vi "oldDataToTDMS.vi"() -> ()   [LabVIEW 2018]
uses:
  PublicSubVI/Class/FileManager/FM.lvclass
  PublicSubVI/Class/ProgressBar/ProgressBar.lvclass
panel:
  in  "Progress":i32(slide) caption="AddPath" scale=0.0..100.0
  out "conversion failure path list":i32(listbox)=-1
  in  "progressCaption":string
  in  "conversion":bool
  in  "path list":i32(listbox)=-1
  in  "add data path":path
  in  "target folder path ( TDMS )":path
  in  "reset":bool
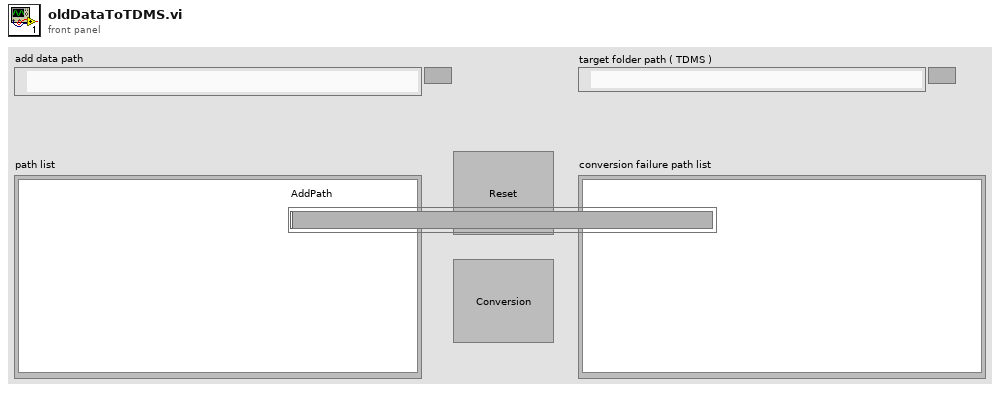
[diagram p1: front panel]
types:
  T1 = cluster{"thisVIRefnum":refnum<vi>, "progressBarRefnum":refnum<vi>, "progressCaption":refnum<vi>}
  T2 = enum16{"open", "open or create", "create or replace", "create", "open (read-only)"}
  T3 = enum16{"open", "replace", "create", "open or create", "replace or create", "replace or create with confirmation"}
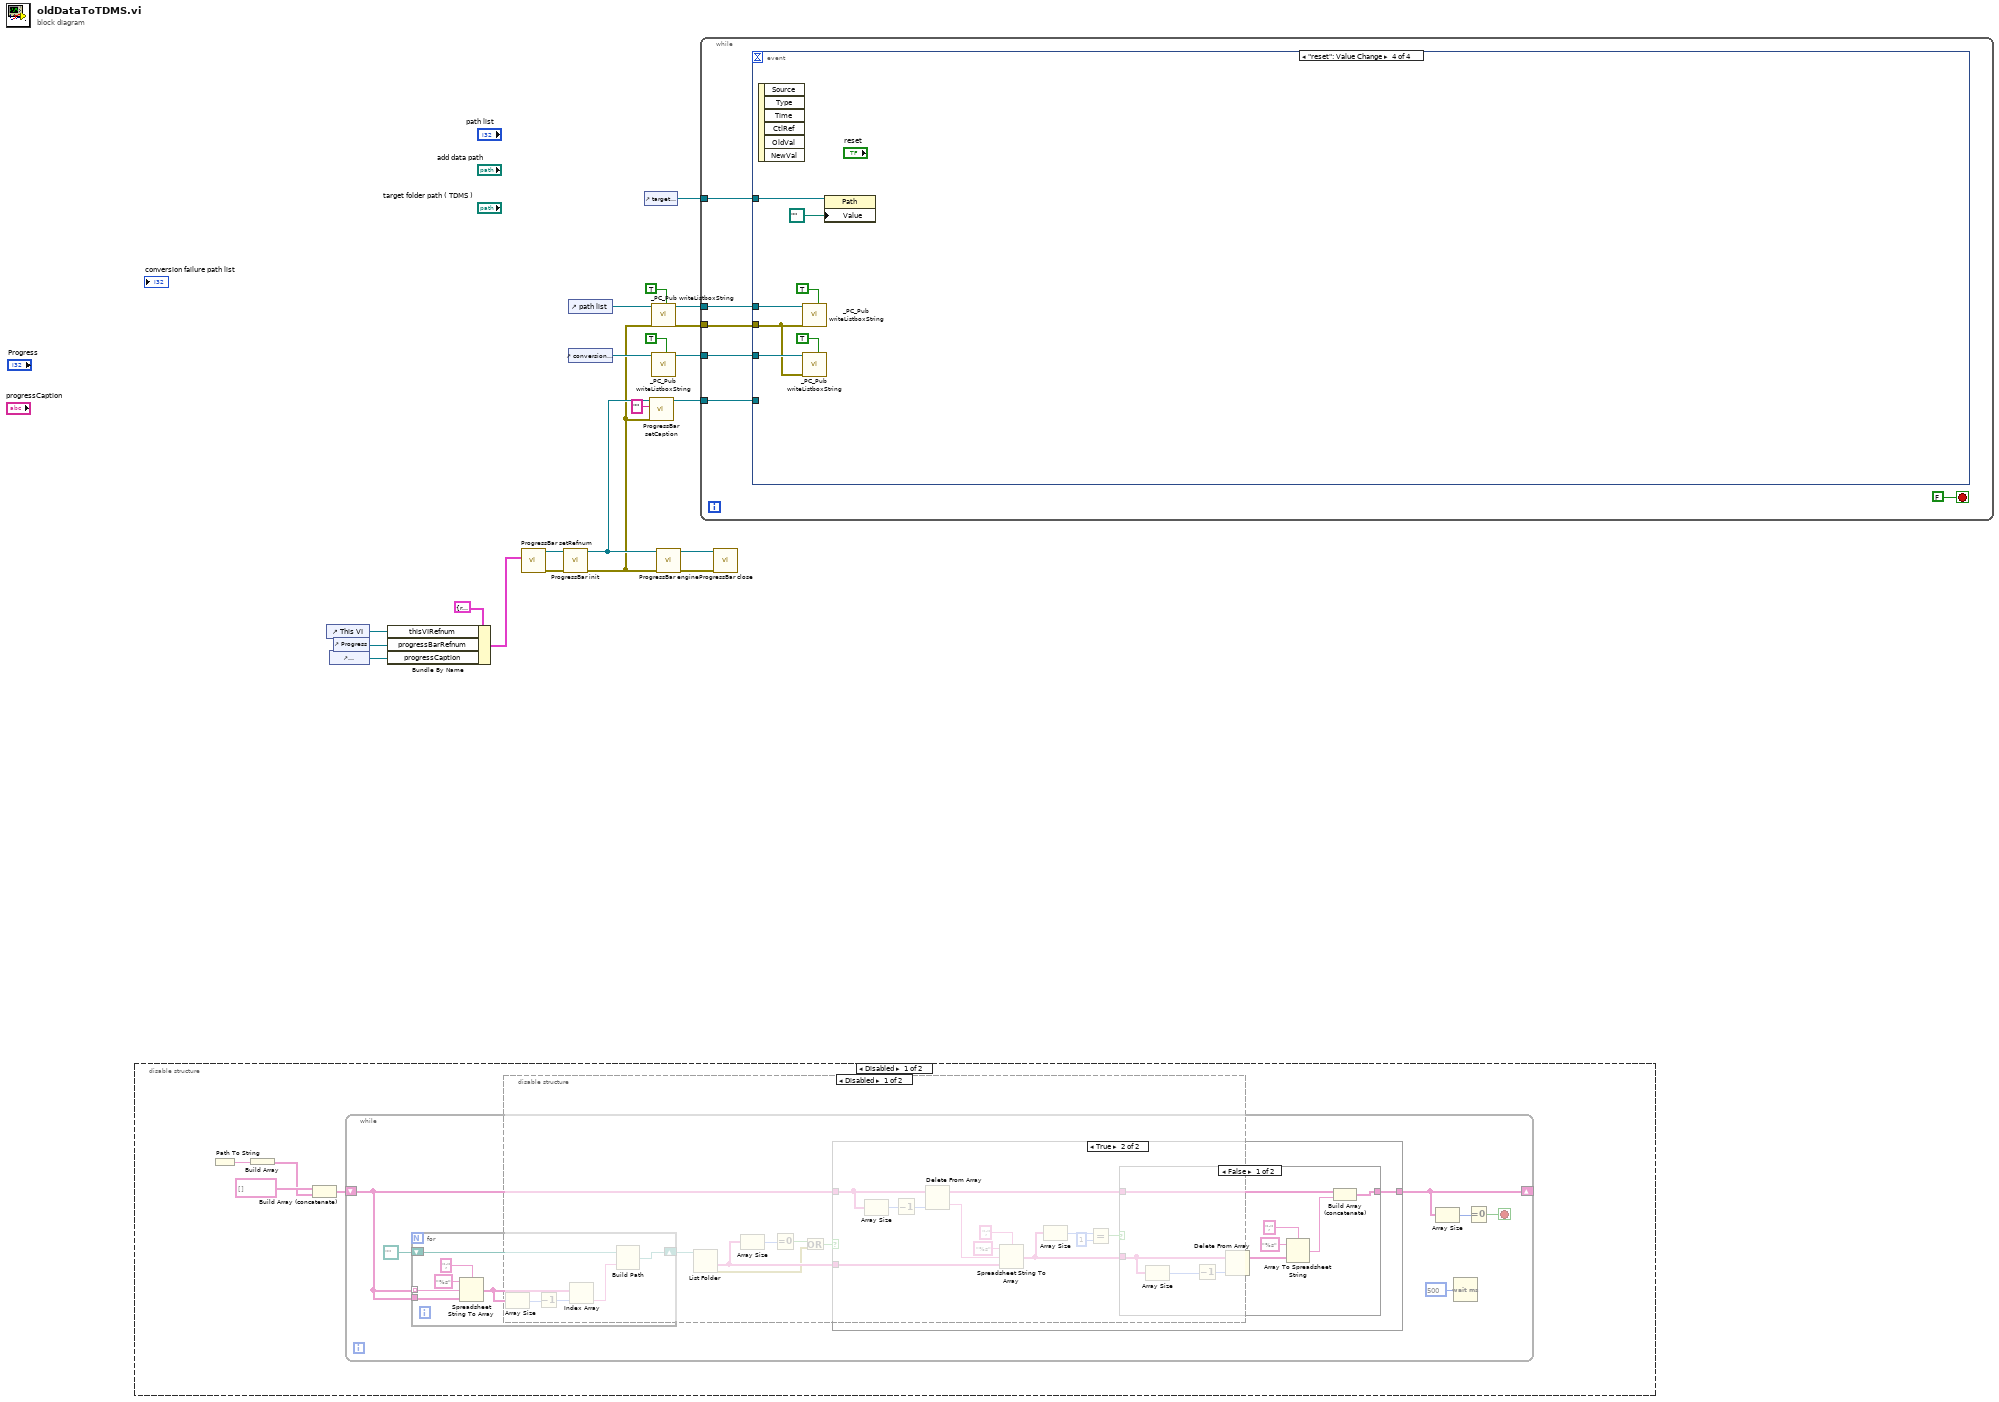
[diagram p0: block diagram]
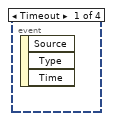
[diagram p2: hidden frame]
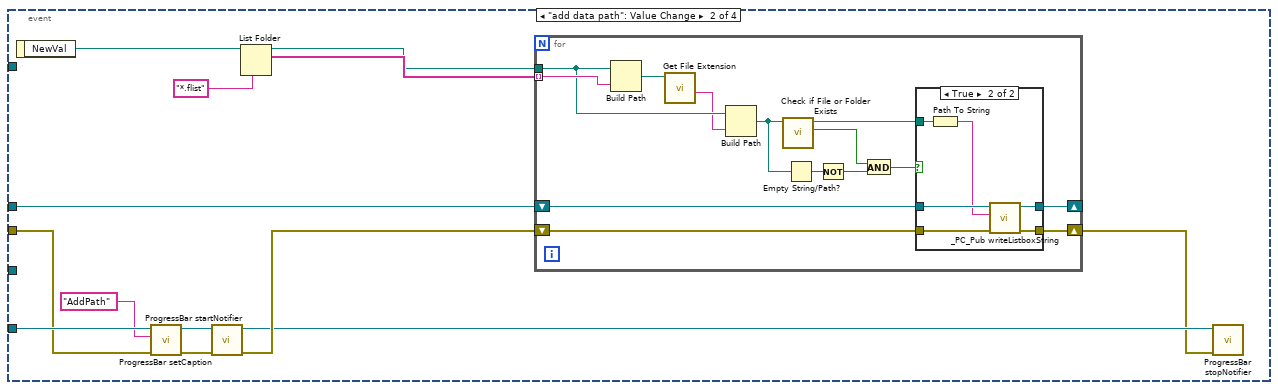
[diagram p3: hidden frame]
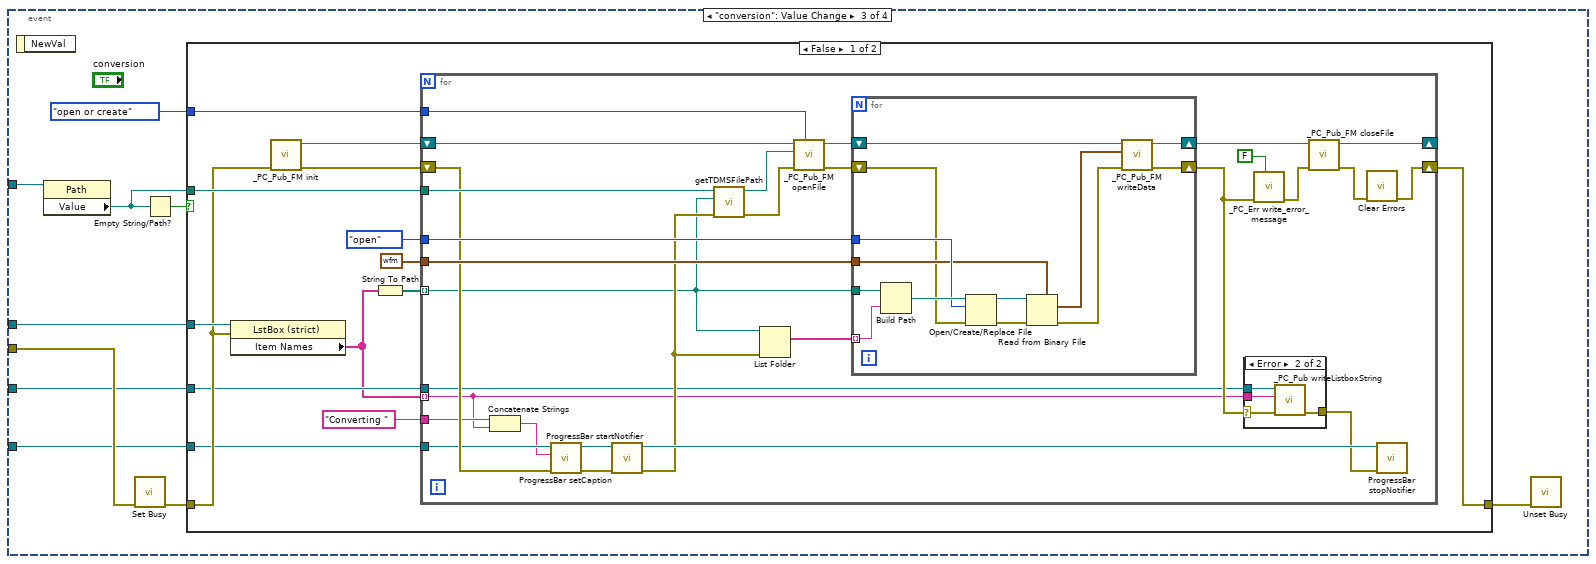
[diagram p5: hidden frame]
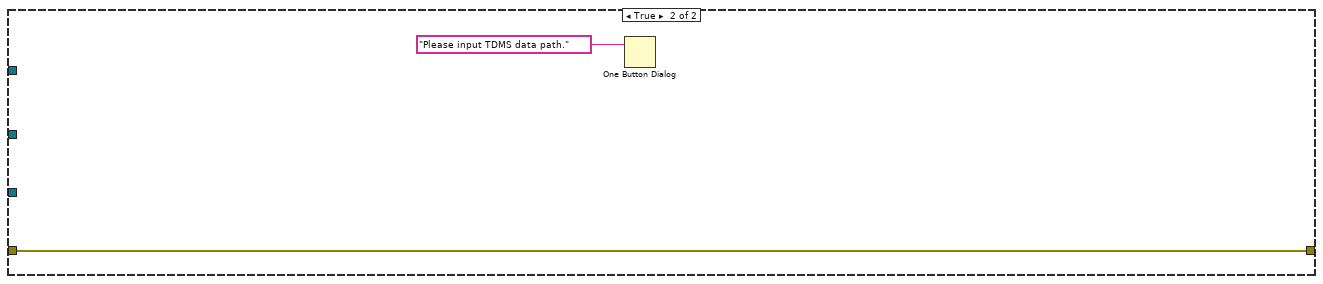
[diagram p7: hidden frame]
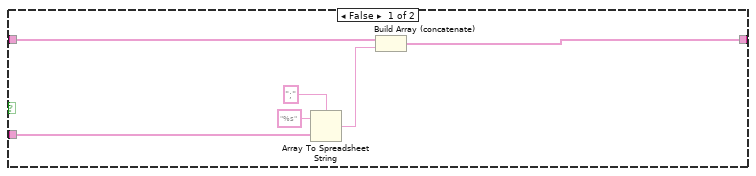
[diagram p8: hidden frame]
diagram:
  n1 = disable-structure shown="Disabled" {
    frame Disabled {
      n2 = Path To String() -> (path=w27:path, string=w25:string)
      n3 = Build Array(w25) -> (w24:string[])
      n4 = Build Array (concatenate)(string[] [], w24) -> (w23:string[])
      n5 = while {
        shift-right: [w35] -> w22
        shift-left: w23 -> [w36]
        i -> [w28]
        stop <- w33 stop-if-true
        n6 = for {
          tunnel: w36 -> [w79] mode=indexing
          shift-right: [w74] -> w37
          shift-left: path "" ("base path") -> [w75]
          tunnel: w36 -> [w78]
          n7 = Spreadsheet String To Array(delimiter (Tab)=";", format string="%s", spreadsheet string=w79, array type (2D Dbl)=w78) -> (array=w73:string[])
          n8 = Array Size(array=w73) -> (size(s)=w72:i32)
          n9 = Decrement(x=w72) -> (x-1=w71:i32)
          n10 = Index Array(array=w73, index=w71) -> (element=w70:string)
          n11 = Build Path(base path=w75, name or relative path=w70) -> (appended path=w74:path)
        }
        n12 = List Folder(path=w37) -> (folder names=w39:string[], error out=w31:errorcluster)  [unwired: 3 in, 2 out]
        n13 = Array Size(array=w39) -> (size(s)=w40:i32)
        n14 = Equal To 0?(x=w40) -> (x = 0?=w32:bool)
        n15 = Or(x=w32, y=w31) -> (x .or. y?=w30:bool)
        n16 = case shown="True" w30 {
          tunnel: w36 -> [w46 w59]
          tunnel: w39 -> [w45 w54]
          tunnel: [w41 w49] -> w35
          frame False {
            n17 = Array To Spreadsheet String(delimiter (Tab)=";", array=w45, 3:"%s" ("format string")) -> (spreadsheet string=w42:string)
            n18 = Build Array (concatenate)(w46, w42) -> (w41:string[])
          }
          frame True {
            n19 = Array Size(array=w59) -> (size(s)=w58:i32)
            n20 = Decrement(x=w58) -> (x-1=w57:i32)
            n21 = Delete From Array(array=w59, index=w57) -> (deleted portion=w56:string, array with subset deleted=w48:string[])  [unwired: 1 in]
            n22 = Spreadsheet String To Array(delimiter (Tab)=";", format string="%s", spreadsheet string=w56, array type (2D Dbl)=w54) -> (array=w47:string[])
            n23 = Array Size(array=w47) -> (size(s)=w52:i32)
            n24 = Equal?(x=w52, y=1) -> (x = y?=w50:bool)
            n25 = case shown="False" w50 {
              tunnel: [w65 w69] -> w49
              tunnel: w48 -> [w60 w69]
              tunnel: w47 -> [w67 _]
              frame False {
                n26 = Array Size(array=w67) -> (size(s)=w68:i32)
                n27 = Decrement(x=w68) -> (x-1=w66:i32)
                n28 = Delete From Array(array=w67, index=w66) -> (array with subset deleted=w64:string[])  [unwired: 1 in, 1 out]
                n29 = Array To Spreadsheet String(delimiter (Tab)=";", array=w64, 3:"%s" ("format string")) -> (spreadsheet string=w61:string)
                n30 = Build Array (concatenate)(w60, w61) -> (w65:string[])
              }
              frame True {
              }
            }
          }
        }
        n31 = Array Size(array=w35) -> (size(s)=w34:i32)
        n32 = Wait (ms)(milliseconds to wait=u32 500) -> ()  [unwired: 1 out]
        n33 = Equal To 0?(x=w34) -> (x = 0?=w33:bool)
      }
    }
    frame Enabled {
    }
  }
  n34 = control-ref of="This VI"() -> (w9:refnum<vi>)
  n35 = control-ref of="progressCaption"() -> (w11:refnum<vi>)
  n36 = control-ref of="Progress"() -> (w10:refnum<vi>)
  n37 = Bundle By Name(cluster=T1 {"thisVIRefnum"=refnum, "progressBarRefnum"=refnum, "progressCaption"=refnum} ("refnum"), "thisVIRefnum"=w9, "progressBarRefnum"=w10, "progressCaption"=w11) -> (w12:T1)
  n38 = disable-structure shown="Disabled" {
    frame Disabled {
    }
    frame Enabled {
    }
  }
  n39 = call "ProgressBar setRefnum.vi"("refnum"=w12) -> ("error out"=w16:errorcluster, "ProgressBar out"=w13:refnum<class "ProgressBar.lvclass">)  [unwired: 9 in]
  n40 = call "ProgressBar init.vi"("error in (no error)"=w16, "ProgressBar in"=w13) -> ("error out"=w2:errorcluster, "ProgressBar out"=w4:refnum<class "ProgressBar.lvclass">)  [unwired: 8 in]
  n41 = control-ref of="path list"() -> (w21:refnum<vi>)
  n42 = control-ref of="conversion failure path list"() -> (w6:refnum<vi>)
  n43 = control-ref of="target folder path ( TDMS )"() -> (w17:refnum<vi>)
  n44 = call "ProgressBar setCaption.vi"("error in (no error)"=w2, "newCaption"="", "ProgressBar in"=w4) -> ("ProgressBar out"=w3:refnum<class "ProgressBar.lvclass">)  [unwired: 7 in, 1 out]
  n45 = call "_PC_Pub writeListboxString.vi"("Reset (F)"=TRUE, "error in (no error)"=w2, "Listbox Ref Input"=w21) -> ("error out"=w18:errorcluster, "Listbox Ref Output"=w19:refnum<vi>)  [unwired: 7 in]
  n46 = call "_PC_Pub writeListboxString.vi"("Reset (F)"=TRUE, "Listbox Ref Input"=w6) -> ("Listbox Ref Output"=w5:refnum<vi>)  [unwired: 8 in, 1 out]
  n47 = call "ProgressBar engine.vi"("error in (no error)"=w2, "ProgressBar in"=w4) -> ("error out"=w15:errorcluster, "ProgressBar out"=w14:refnum<class "ProgressBar.lvclass">)  [unwired: 8 in]
  n48 = while {
    tunnel: w19 -> [w85]
    tunnel: w18 -> [w84]
    tunnel: w17 -> [w82]
    tunnel: w3 -> [w81]
    tunnel: w5 -> [w80]
    stop <- FALSE stop-if-true
    n49 = event shown="[3] \"reset\": Value Change" {
      selector: _ -> [_ _ _ _]
      dyn-events: _ -> [_ _ _ _]
      timeout: _ -> [_ _ _ _]
      tunnel: w85 -> [_ w94 w127 w198]
      tunnel: w84 -> [_ w88 w125 w196]
      tunnel: w82 -> [_ _ w130 w195]
      tunnel: w81 -> [_ w90 w122 _]
      tunnel: w80 -> [_ _ w121 w197]
      event Timeout {
        n50 = event-data() -> ()  [unwired: 1 in, 3 out]
      }
      event "add data path": Value Change {
        n51 = event-data() -> ("NewVal"=w98:path)  [unwired: 1 in]
        n52 = call "ProgressBar setCaption.vi"("error in (no error)"=w88, "newCaption"="AddPath", "ProgressBar in"=w90) -> ("error out"=w91:errorcluster, "ProgressBar out"=w92:refnum<class "ProgressBar.lvclass">)  [unwired: 7 in]
        n53 = call "ProgressBar startNotifier.vi"("error in (no error)"=w91, "ProgressBar in"=w92) -> ("error out"=w93:errorcluster, "ProgressBar out"=w87:refnum<class "ProgressBar.lvclass">)  [unwired: 8 in]
        n54 = List Folder(path=w98, pattern="*.flist") -> (path out=w95:path, filenames=w96:string[])  [unwired: 2 in, 2 out]
        n55 = for {
          tunnel: w96 -> [w112] mode=indexing
          tunnel: w95 -> [w110]
          shift-right: [w100] -> w86
          shift-left: w93 -> [w99]
          shift-right: [w101] -> _
          shift-left: w94 -> [w102]
          n56 = Build Path(base path=w110, name or relative path=w112) -> (appended path=w111:path)
          n57 = call <vilib>:"Get File Extension.vi"("file"=w111) -> ("filename without extension"=w109:string)  [unwired: 6 in, 4 out]
          n58 = Build Path(base path=w110, name or relative path=w109) -> (appended path=w108:path)
          n59 = call <vilib>:"Check if File or Folder Exists.vi"("path"=w108) -> ("file or folder exists?"=w106:bool, "dup path"=w103:path)  [unwired: 8 in, 1 out]
          n60 = Empty String/Path?(string/path=w108) -> (empty?=w107:bool)
          n61 = Not(x=w107) -> (.not. x?=w105:bool)
          n62 = And(x=w106, y=w105) -> (x .and. y?=w104:bool)
          n63 = case shown="True" w104 {
            tunnel: w103 -> [_ w120]
            tunnel: w102 -> [w114 w119]
            tunnel: [w114 w118] -> w101
            tunnel: [w113 w117] -> w100
            tunnel: w99 -> [w113 w116]
            frame False {
            }
            frame True {
              n64 = Path To String(path=w120) -> (string=w115:string)
              n65 = call "_PC_Pub writeListboxString.vi"("error in (no error)"=w116, "update_Str"=w115, "Listbox Ref Input"=w119) -> ("error out"=w117:errorcluster, "Listbox Ref Output"=w118:refnum<vi>)  [unwired: 7 in]
            }
          }
        }
        n66 = call "ProgressBar stopNotifier.vi"("error in (no error)"=w86, "ProgressBar in"=w87) -> ()  [unwired: 8 in, 2 out]
      }
      event "conversion": Value Change {
        n67 = event-data() -> ()  [unwired: 1 in, 1 out]
        n68 = property class="Path"(reference=w130) -> ("Value"=w128:path)  [unwired: 1 in, 2 out]
        n69 = call <vilib>:"Set Busy.vi"("error in (no error)"=w125) -> ("error out"=w124:errorcluster)  [unwired: 9 in, 1 out]
        n70 = Empty String/Path?(string/path=w128) -> (empty?=w129:bool)
        n71 = case shown="False" w129 {
          tunnel: w128 -> [w140 _]
          tunnel: w127 -> [w144 _]
          tunnel: T2."open or create" ("operation (0:open)") -> [w137 _]
          tunnel: w124 -> [w136 w192]
          tunnel: [w133 w192] -> w123
          tunnel: w122 -> [w132 _]
          tunnel: w121 -> [w135 _]
          frame False {
            n72 = property class="LstBox (strict)"(reference=w144, error in=w136) -> ("Item Names"=w134:string[])  [unwired: 2 out]
            n73 = call "_PC_Pub_FM init.vi"("error in (no error)"=w136) -> ("error out"=w138:errorcluster, "FM out"=w139:refnum<class "FM.lvclass">)  [unwired: 9 in]
            n74 = String To Path(string=w134) -> (path=w143:path[])
            n75 = for {
              tunnel: w143 -> [w155] mode=indexing
              tunnel: T3."open" ("operation (0:open)") -> [w172]
              tunnel: waveform(sgl) {"t0"=timestamp(0 s since 1904-01-01), "dt"=1.0, "Y"=[]} ("Spectrum data in") -> [w171]
              tunnel: w140 -> [w165]
              tunnel: w137 -> [w170]
              shift-right: [w167] -> _
              shift-left: w139 -> [w169]
              shift-right: [w149] -> w133
              shift-left: w138 -> [w160]
              tunnel: w135 -> [w153]
              tunnel: w134 -> [w146] mode=indexing
              tunnel: w132 -> [w148]
              tunnel: "Converting " -> [w147]
              n76 = Concatenate Strings(w147, w146) -> (w145:string)
              n77 = call "ProgressBar setCaption.vi"("error in (no error)"=w160, "newCaption"=w145, "ProgressBar in"=w148) -> ("error out"=w162:errorcluster, "ProgressBar out"=w161:refnum<class "ProgressBar.lvclass">)  [unwired: 7 in]
              n78 = call "ProgressBar startNotifier.vi"("error in (no error)"=w162, "ProgressBar in"=w161) -> ("error out"=w156:errorcluster, "ProgressBar out"=w158:refnum<class "ProgressBar.lvclass">)  [unwired: 8 in]
              n79 = call "getTDMSFilePath.vi"("error in (no error)"=w156, "sourceFolder"=w155, "moveFolder"=w165) -> ("error out"=w164:errorcluster, "tdmsFilePath"=w163:path)  [unwired: 7 in]
              n80 = List Folder(path=w155, error in=w156) -> (filenames=w173:string[])  [unwired: 2 in, 3 out]
              n81 = call "_PC_Pub_FM openFile.vi"("operation (0:open)"=w170, "error in (no error)"=w164, "openPath"=w163, "FM in"=w169) -> ("error out"=w157:errorcluster, "FM out"=w166:refnum<class "FM.lvclass">)  [unwired: 6 in]
              n82 = for {
                tunnel: w155 -> [w191]
                tunnel: w173 -> [w190] mode=indexing
                tunnel: w172 -> [w186]
                tunnel: w171 -> [w185]
                shift-right: [w182] -> w168
                shift-left: w166 -> [w184]
                shift-right: [w181] -> w154
                shift-left: w157 -> [w180]
                n83 = Build Path(base path=w191, name or relative path=w190) -> (appended path=w187:path)
                n84 = Open/Create/Replace File(file path (use dialog)=w187, error in=w180, operation (0:open)=w186) -> (refnum out=w189:refnum<file>, error out=w188:errorcluster)  [unwired: 3 in, 1 out]
                n85 = Read from Binary File(5:w185, 8:w188, 11:w189) -> (0:w179:errorcluster, 2:w183:waveform(sgl))  [unwired: 3 in, 2 out]
                n86 = call "_PC_Pub_FM writeData.vi"("error in (no error)"=w179, "element"=w183, "FM in"=w184) -> ("error out"=w181:errorcluster, "FM out"=w182:refnum<class "FM.lvclass">)  [unwired: 7 in]
              }
              n87 = case shown="Error" w154 {
                selector: w154 -> [w174 w176]
                tunnel: w153 -> [_ w178]
                tunnel: w146 -> [_ w177]
                tunnel: [w174 w175] -> w152
                frame No Error {
                }
                frame Error {
                  n88 = call "_PC_Pub writeListboxString.vi"("error in (no error)"=w176, "update_Str"=w177, "Listbox Ref Input"=w178) -> ("error out"=w175:errorcluster)  [unwired: 7 in, 1 out]
                }
              }
              n89 = call "_PC_Err write_error_message.vi"("show msg( T )"=FALSE, "error in"=w154) -> ("error out"=w159:errorcluster)  [unwired: 9 in]
              n90 = call "_PC_Pub_FM closeFile.vi"("error in (no error)"=w159, "FM in"=w168) -> ("error out"=w150:errorcluster, "FM out"=w167:refnum<class "FM.lvclass">)  [unwired: 7 in, 1 out]
              n91 = call <vilib>:"Clear Errors.vi"("error in (no error)"=w150) -> ("error out"=w149:errorcluster)  [unwired: 5 in, 1 out]
              n92 = call "ProgressBar stopNotifier.vi"("error in (no error)"=w152, "ProgressBar in"=w158) -> ()  [unwired: 8 in, 2 out]
            }
          }
          frame True {
            n93 = One Button Dialog(message="Please input TDMS data path.") -> ()  [unwired: 1 in, 1 out]
          }
        }
        n94 = call <vilib>:"Unset Busy.vi"("error in (no error)"=w123) -> ()  [unwired: 10 in, 1 out]
      }
      event "reset": Value Change {
        n95 = event-data() -> ()  [unwired: 1 in, 6 out]
        n96 = call "_PC_Pub writeListboxString.vi"("Reset (F)"=TRUE, "error in (no error)"=w196, "Listbox Ref Input"=w198) -> ()  [unwired: 7 in, 2 out]
        n97 = call "_PC_Pub writeListboxString.vi"("Reset (F)"=TRUE, "error in (no error)"=w196, "Listbox Ref Input"=w197) -> ()  [unwired: 7 in, 2 out]
        n98 = property class="Path"(reference=w195, "Value"=path "") -> ()  [unwired: 1 in, 2 out]
      }
    }
  }
  n99 = call "ProgressBar close.vi"("error in (no error)"=w15, "ProgressBar in"=w14) -> ()  [unwired: 8 in, 2 out]
